vi "FAST-PS Example Voltage Loop Control.vi"() -> ()   [LabVIEW 2025, in "CAENels FAST-PS.lvlib"]
doc: "When the example is executed, it sets the FAST-PS to CV mode and updates the set-point 10 times per second."
uses:
  CAENels FAST-PS.lvlib
panel:
  out "Regulation mode":bool
  out "Fault condition":bool
  out "ON/OFF":bool
  in  "IP address":string="192.168.0.10"
  out "Output Voltage Chart":dbl(graph)
  in  "Stop Button":bool
  in  "Voltage Setpoint":dbl
  out "Output Voltage":string
  out "Output Current":string
  out "Module Status":string
  # "0: CC\n1: CV"
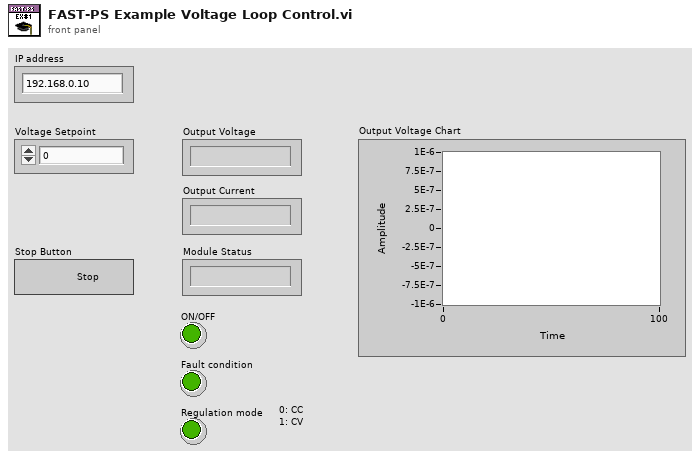
[diagram p1: front panel]
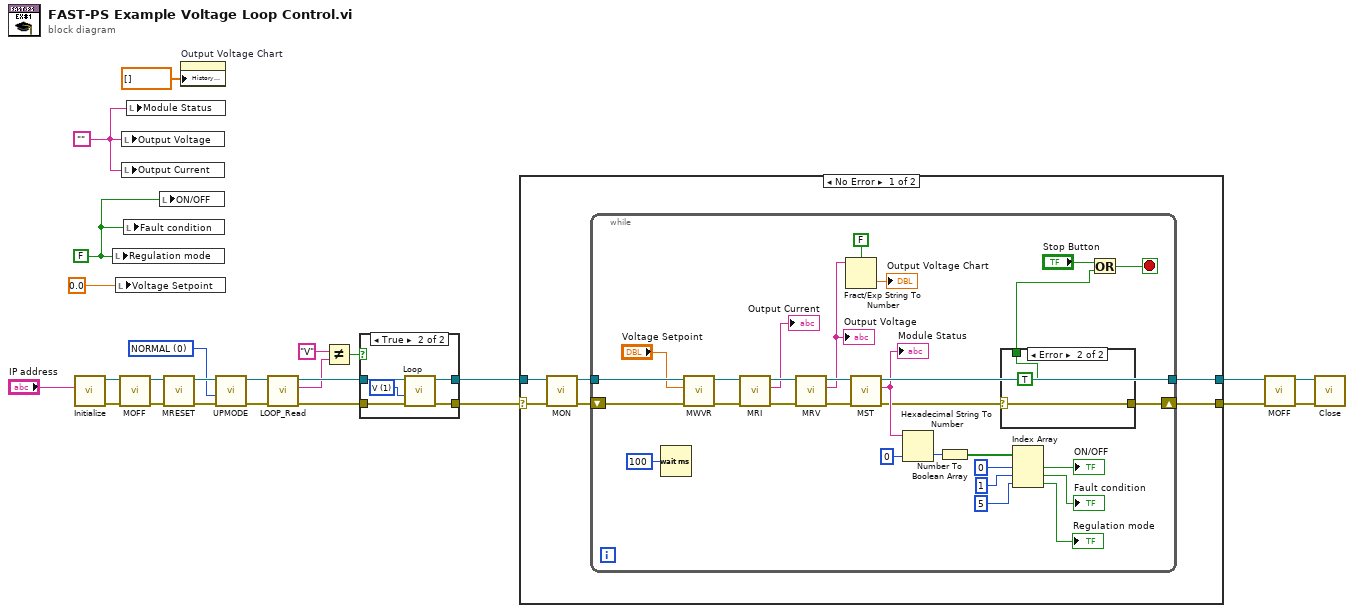
[diagram p0: block diagram]
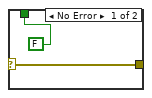
[diagram p2: hidden frame]
diagram:
  w3 = ""
  w4 = FALSE ("Regulation mode")
  w14 = 0 items=["NORMAL", "ANALOG"] ("UPMODE")
  n1 = call "Initialize.vi"("IP address"="IP address") -> ("error out"=w8:errorcluster, "connection ID"=w10:refnum<k5>)  [unwired: 5 in]
  n2 = local write "Regulation mode"(w4) -> ()
  n3 = local write "Voltage Setpoint"(0.0 ("Voltage Setpoint")) -> ()
  n4 = call "MOFF.vi"("error in (no error)"=w8, "connection ID"=w10) -> ("error out"=w7:errorcluster, "connection ID out"=w9:refnum<k5>)  [unwired: 4 in]
  n5 = local write "Output Voltage"(w3) -> ()
  n6 = local write "Output Current"(w3) -> ()
  n7 = local write "Fault condition"(w4) -> ()
  n8 = local write "Module Status"(w3) -> ()
  n9 = local write "ON/OFF"(w4) -> ()
  n10 = call "MRESET.vi"("error in (no error)"=w7, "connection ID"=w9) -> ("error out"=w19:errorcluster, "connection ID out"=w20:refnum<k5>)  [unwired: 4 in]
  n11 = property on="Output Voltage Chart" class="WFChart (strict)"("History Data"=dbl[] []) -> ()  [unwired: 2 in, 2 out]
  n12 = call "UPMODE.vi"("error in (no error)"=w19, "UPMODE"=w14, "connection ID"=w20) -> ("error out"=w11:errorcluster, "connection ID out"=w12:refnum<k5>)  [unwired: 3 in]
  n13 = call "LOOP_Read.vi"("error in (no error)"=w11, "connection ID"=w12) -> ("error out"=w23:errorcluster, "LOOP response"=w22:string, "connection ID out"=w24:refnum<k5>)  [unwired: 3 in]
  n14 = Not Equal?(x="V" ("string (\"\")"), y=w22) -> (x != y?=w21:bool)
  n15 = case shown="True" w21 {
    tunnel: w24 -> [w27 w32]
    tunnel: w23 -> [w26 w31]
    tunnel: [w27 w30] -> w6
    tunnel: [w26 w29] -> w1
    frame False {
    }
    frame True {
      w28 = 1 items=["I", "V"] ("UPMODE")
      n16 = call "Loop.vi"("error in (no error)"=w31, "LOOP"=w28, "connection ID"=w32) -> ("error out"=w29:errorcluster, "connection ID out"=w30:refnum<k5>)  [unwired: 3 in]
    }
  }
  n17 = case shown="No Error" w1 {
    selector: w1 -> [w33 w73]
    tunnel: [w38 w73] -> w16
    tunnel: [w37 w74] -> w15
    tunnel: w6 -> [w34 w74]
    frame No Error {
      n18 = call "MON.vi"("error in (no error)"=w33, "connection ID"=w34) -> ("error out"=w36:errorcluster, "connection ID out"=w35:refnum<k5>)  [unwired: 4 in]
      n19 = while {
        tunnel: [w68] -> w37
        tunnel: w35 -> [w62]
        shift-right: [w42] -> w38
        shift-left: w36 -> [w60]
        stop <- w40 stop-if-true
        n20 = Wait (ms)(milliseconds to wait=u32 100) -> ()  [unwired: 1 out]
        n21 = call "MWVR.vi"("error in (no error)"=w60, "voltage"="Voltage Setpoint", "connection ID"=w62) -> ("error out"=w59:errorcluster, "connection ID out"=w61:refnum<k5>)  [unwired: 3 in]
        n22 = call "MRI.vi"("error in (no error)"=w59, "connection ID"=w61) -> ("error out"=w66:errorcluster, "current"=→"Output Current":string, "connection ID out"=w67:refnum<k5>)  [unwired: 3 in]
        n23 = call "MRV.vi"("error in (no error)"=w66, "connection ID"=w67) -> ("error out"=w64:errorcluster, "voltage"=w55:string, "connection ID out"=w65:refnum<k5>)  [unwired: 3 in]
        "Output Voltage" <- w55
        n24 = Fract/Exp String To Number(use system decimal point (T)=FALSE, string=w55) -> (number=→"Output Voltage Chart":dbl)  [unwired: 2 in, 1 out]
        n25 = call "MST.vi"("error in (no error)"=w64, "connection ID"=w65) -> ("error out"=w43:errorcluster, "MST response"=w53:string, "connection ID out"=w68:refnum<k5>)  [unwired: 3 in]
        "Module Status" <- w53
        n26 = Hexadecimal String To Number(string=w53, default (0uL)=u32 0 ("default (0 U32)")) -> (number=w51:u32)  [unwired: 1 in, 1 out]
        n27 = Number To Boolean Array(number=w51) -> (Boolean array=w50:bool[])
        n28 = case shown="Error" w43 {
          selector: w43 -> [w70 w71]
          tunnel: [w70 w71] -> w42
          tunnel: [FALSE TRUE] -> w39
          frame No Error {
          }
          frame Error {
          }
        }
        n29 = Index Array(array=w50, index #1=0 ("index"), index #2=1 ("index"), index #3=5 ("index")) -> (element #1=→"ON/OFF":bool, element #2=→"Fault condition":bool, element #3=→"Regulation mode":bool)
        n30 = Or(x="Stop Button", y=w39) -> (x .or. y?=w40:bool)
      }
    }
    frame Error {
    }
  }
  n31 = call "MOFF.vi"("error in (no error)"=w16, "connection ID"=w15) -> ("error out"=w17:errorcluster, "connection ID out"=w18:refnum<k5>)  [unwired: 4 in]
  n32 = call "Close.vi"("error in (no error)"=w17, "connection ID"=w18) -> ()  [unwired: 5 in, 1 out]
